vi "Resource Editor.vi"(7 "Load from Initial Path (F)":bool, 10 "Initial Resources":T1, 11 "Path":path) -> (2 "Final Resources":T1)   [LabVIEW 2023]
doc: "Edits several types of LabVIEW files at a low level, including VI's.\n\nCan also be used as a dialog subVI for editing resource clusters."
uses:
  Resource Manipulation/Resource Array.ctl
  Resource Manipulation/Resource.ctl
  CTLs/Resource Editor Internal Commands Enum.ctl
  Resource Manipulation.lvlib
panel:
  out "Initial Resources 2":T1
  in  "Delete":bool
  in  "Add":bool
  in  "Name":string
  in  "Type":string
  in  "ID":i32
  in  "Export":bool
  in  "Import":bool
  in  "Paste":bool
  in  "Copy":bool
  in  "XML":bool
  in  "Fix MD5":bool
  in  "File type":string
  in  "Data":string
  in  "Hex view":bool
  in  "Save":bool
  in  "Load":bool
  in  "Resources":i32(listbox)=-1
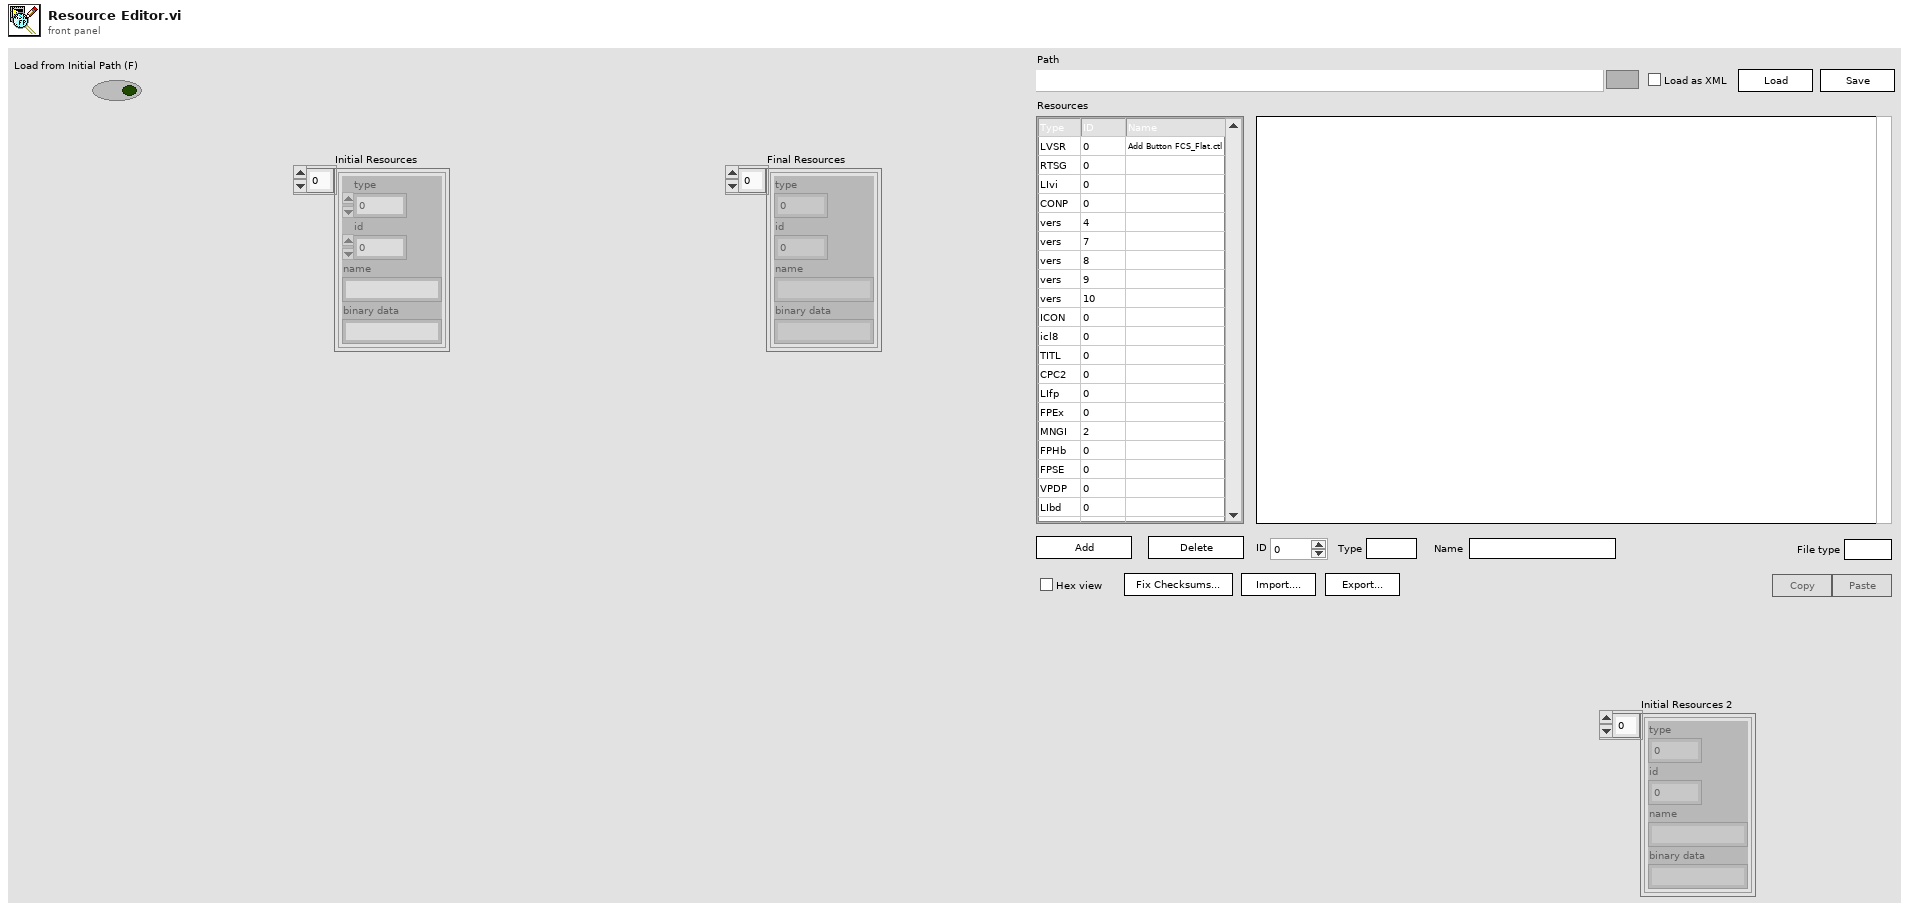
[diagram p1: front panel]
types:
  T1 = typedef "Resource Manipulation.lvlib/Resource Array.ctl" = T2[]
  T2 = typedef "Resource Manipulation.lvlib/Resource.ctl" = cluster{"type":u32, "id":i32, "name":string, "binary data":string}
  T3 = typedef "Resource Editor Internal Commands Enum.ctl" = enum16{"Refresh Resource List", "Load from Path"}
  T4 = enum8{"Enabled", "Disabled", "Disabled and Grayed Out"}
  T5 = enum16{"Left Button", "Center Button", "Right Button", "Window Close"}
  T6 = enum16{"open", "replace", "create", "open or create", "replace or create", "replace or create with confirmation"}
  T7 = typedef "Resource Manipulation.lvlib/Terminal Counts.ctl" = cluster{"Numbers":u32, "Strings":u32, "Paths":u32}
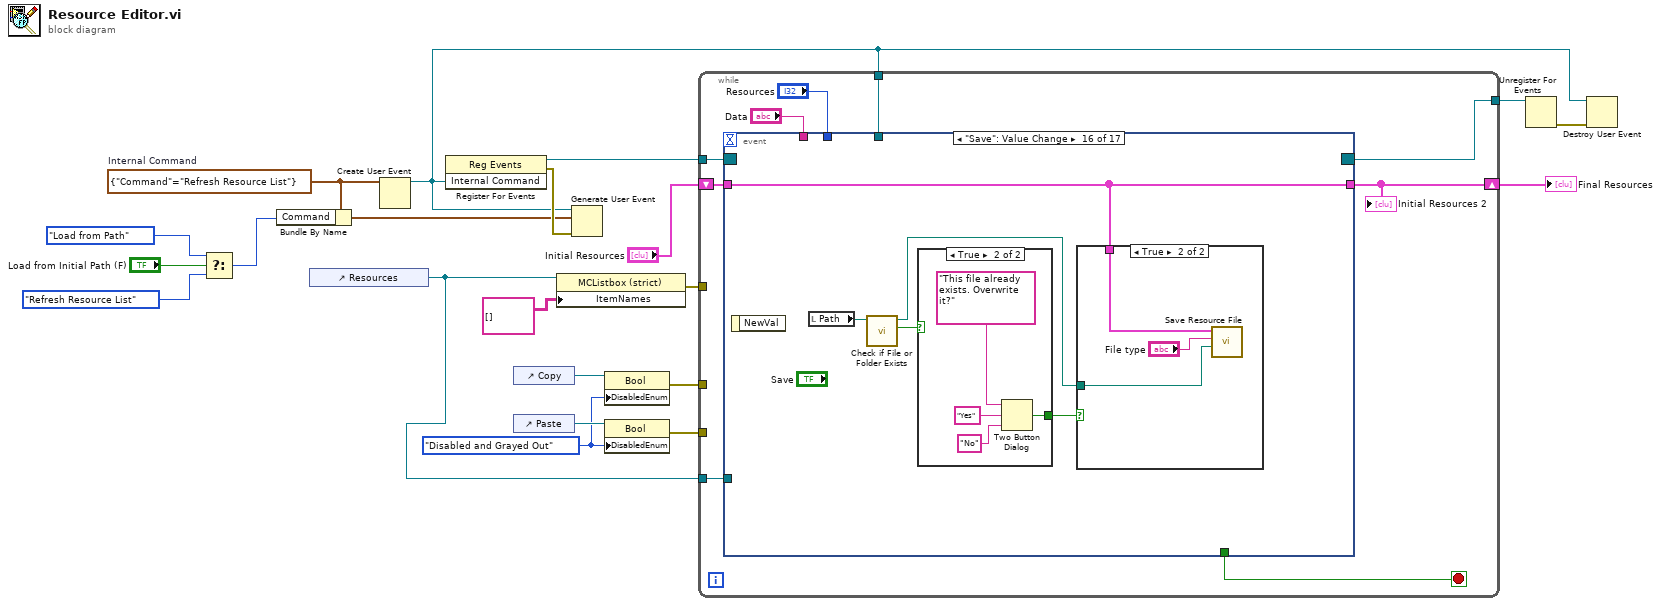
[diagram p0: block diagram]
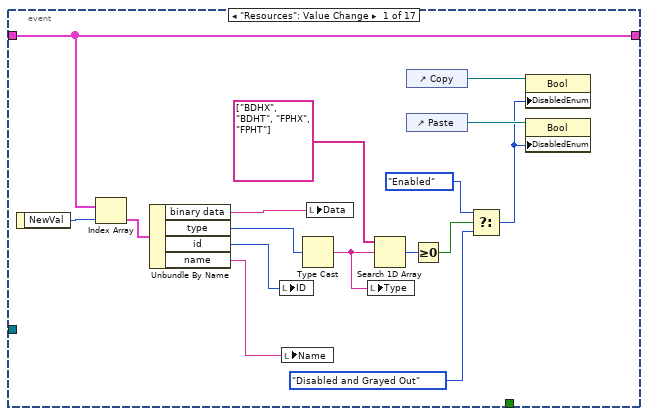
[diagram p2: hidden frame]
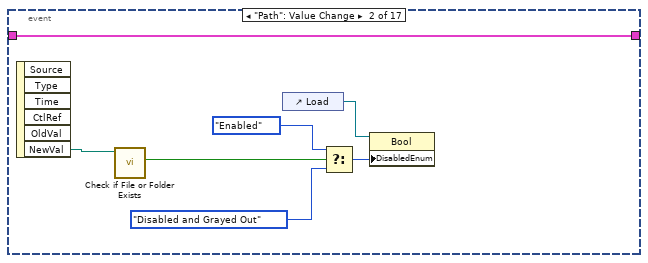
[diagram p3: hidden frame]
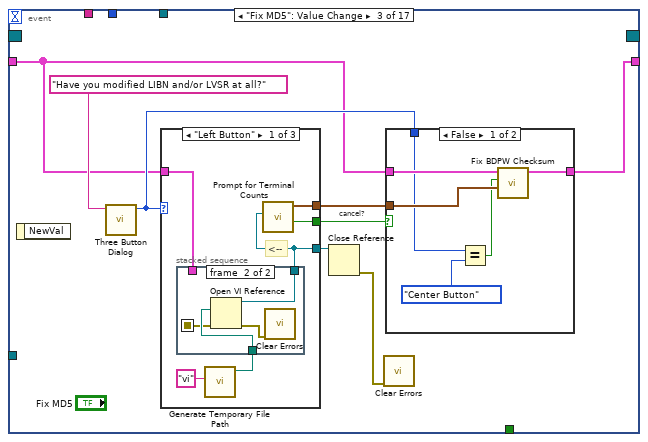
[diagram p4: hidden frame]
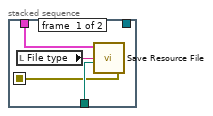
[diagram p5: hidden frame]
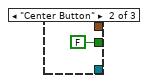
[diagram p6: hidden frame]
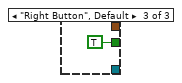
[diagram p7: hidden frame]
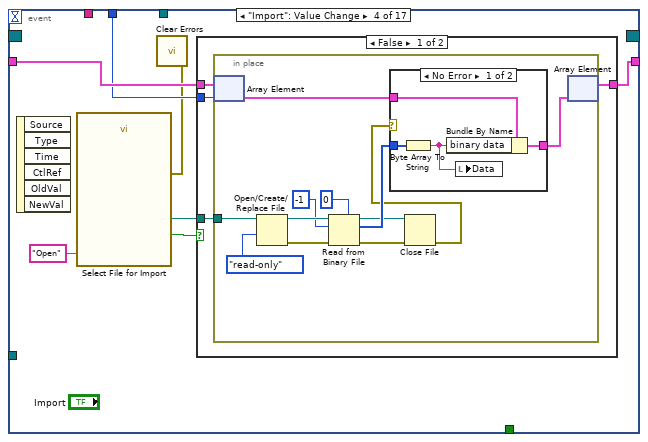
[diagram p9: hidden frame]
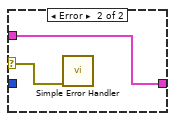
[diagram p10: hidden frame]
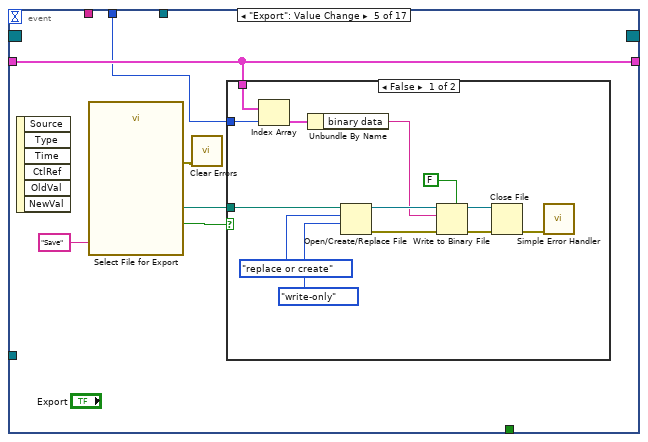
[diagram p12: hidden frame]
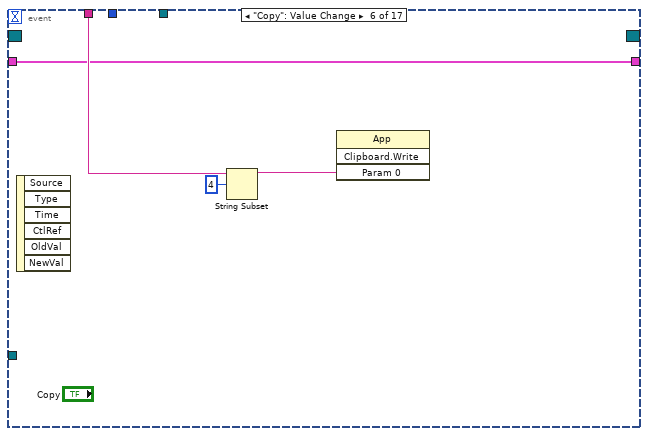
[diagram p14: hidden frame]
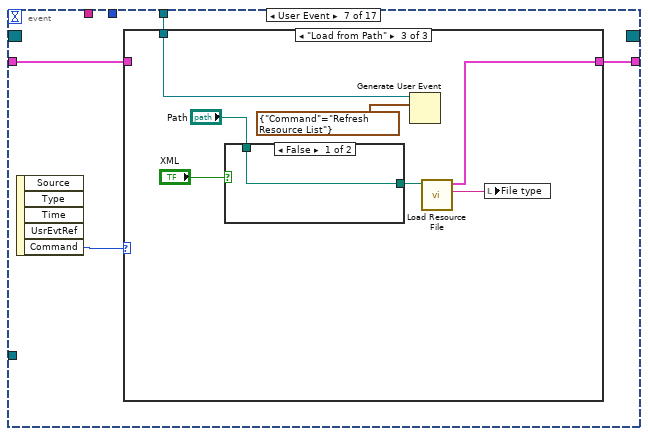
[diagram p15: hidden frame]
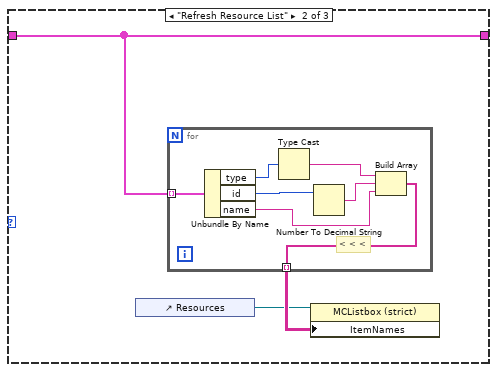
[diagram p17: hidden frame]
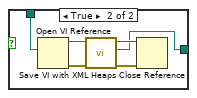
[diagram p18: hidden frame]
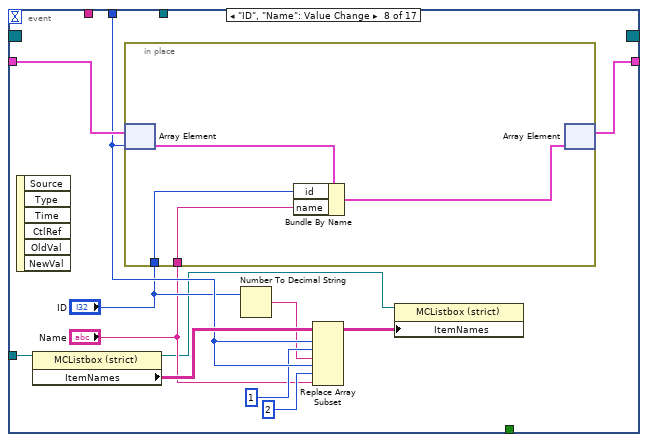
[diagram p19: hidden frame]
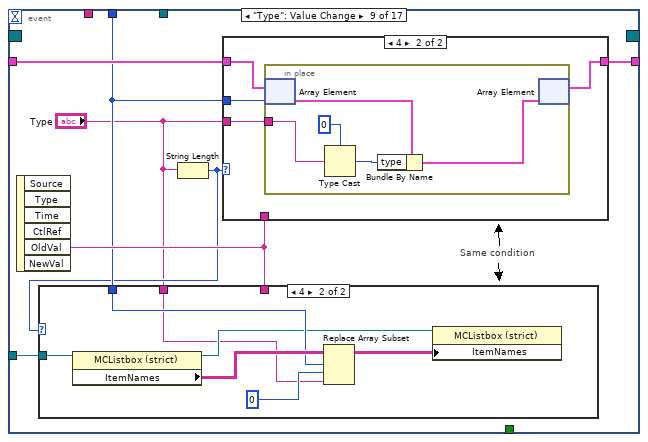
[diagram p20: hidden frame]
diagram:
  w6 = cluster{"Command":T3} {"Command"=enum."Refresh Resource List"}  # Internal Command
  w16 = T4."Disabled and Grayed Out" ("Disabled")
  n1 = Select(t=Resource_Editor_Internal_Commands_Enum."Load from Path" ("Command"), s="Load from Initial Path (F)", f=Resource_Editor_Internal_Commands_Enum."Refresh Resource List" ("Command")) -> (s? t:f=w1:T3)
  n2 = Bundle By Name(cluster=w6, "Command"=w1) -> (w5:cluster{"Command":T3})
  n3 = control-ref of="Resources"() -> (w13:refnum<vi>)
  n4 = Create User Event(user event datatype=w6) -> (user event=w7:refnum<user-event>)  [unwired: 1 in, 1 out]
  n5 = register-events(w7) -> (reference out=w8:refnum<event-registration>, error out=w9:errorcluster)  [unwired: 2 in]
  n6 = control-ref of="Copy"() -> (w18:refnum<vi>)
  n7 = control-ref of="Paste"() -> (w17:refnum<vi>)
  n8 = property class="MCListbox (strict)"(reference=w13, "ItemNames"=string[][] [] ("Item Names")) -> (error out=w20:errorcluster)  [unwired: 1 in, 1 out]
  n9 = Generate User Event(user event=w7, event data cluster=w5, error in=w9) -> ()  [unwired: 1 in, 2 out]
  n10 = property class="Bool"(reference=w18, "DisabledEnum"=w16) -> (error out=w15:errorcluster)  [unwired: 1 in, 1 out]
  n11 = property class="Bool"(reference=w17, "DisabledEnum"=w16) -> (error out=w14:errorcluster)  [unwired: 1 in, 1 out]
  n12 = while {
    shift-right: [w29] -> w12
    shift-left: "Initial Resources" -> [w30]
    tunnel: w20 -> [_]
    tunnel: w15 -> [_]
    tunnel: w14 -> [_]
    tunnel: w13 -> [w25]
    tunnel: w8 -> [w24]
    tunnel: w7 -> [w23]
    tunnel: [w22] -> w11
    stop <- w28 stop-if-true
    n13 = event shown="[15] \"Save\": Value Change" {
      selector: w24 -> [_ _ _ _ _ _ _ _ _ _ _ _ _ _ _ _ _]
      dyn-events: [_ _ _ _ _ _ _ _ _ _ _ _ _ _ _ _ _] -> w22
      timeout: _ -> [_ _ _ _ _ _ _ _ _ _ _ _ _ _ _ _ _]
      tunnel: w30 -> [w44 w47 w57 w91 w120 w136 w139 w178 w189 w216 w232 w241 w246 w253 w260 w265 w274]
      tunnel: [w44 w47 w61 w89 w120 w136 w140 w177 w188 w214 w230 w241 w246 w251 w258 w265 w274] -> w29
      tunnel: [_ _ _ _ _ _ _ _ _ _ _ _ _ _ _ _ w275] -> w28
      tunnel: "Data" -> [_ _ _ _ _ w137 _ _ _ _ _ _ _ _ _ _ _]
      tunnel: "Resources" -> [_ _ _ w90 w117 _ _ w175 w185 w215 w229 _ _ w247 w259 _ _]
      tunnel: w25 -> [_ _ _ _ _ _ _ w168 w187 _ _ _ _ _ _ _ _]
      tunnel: w23 -> [_ _ _ _ _ _ w138 _ _ _ _ _ w244 _ w257 _ _]
      event "Resources": Value Change {
        n14 = event-data() -> ("NewVal"=w46:i32)  [unwired: 1 in]
        n15 = Index Array(array=w44, index=w46) -> (element=w45:T2)
        n16 = Unbundle By Name(w45) -> ("binary data"=w43:string, "type"=w42:u32, "id"=w33:i32, "name"=w32:string)
        n17 = local write "ID"(w33) -> ()
        n18 = local write "Name"(w32) -> ()
        n19 = Type Cast(x=w42) -> (*(type *) &x=w31:string)  [unwired: 1 in]
        n20 = local write "Data"(w43) -> ()
        n21 = local write "Type"(w31) -> ()
        n22 = Search 1D Array(1D array=string[] ["BDHX", "BDHT", "FPHX", "FPHT"], element=w31) -> (index of element=w38:i32)  [unwired: 1 in]
        n23 = control-ref of="Copy"() -> (w40:refnum<vi>)
        n24 = control-ref of="Paste"() -> (w39:refnum<vi>)
        n25 = Greater Or Equal To 0?(x=w38) -> (x >= 0?=w37:bool)
        n26 = Select(t=T4."Enabled" ("Disabled"), s=w37, f=T4."Disabled and Grayed Out" ("Disabled")) -> (s? t:f=w34:T4)
        n27 = property class="Bool"(reference=w40, "DisabledEnum"=w34) -> ()  [unwired: 1 in, 2 out]
        n28 = property class="Bool"(reference=w39, "DisabledEnum"=w34) -> ()  [unwired: 1 in, 2 out]
      }
      event "Path": Value Change {
        n29 = event-data() -> ("NewVal"=w53:path)  [unwired: 1 in, 5 out]
        n30 = call <vilib>:"Check if File or Folder Exists.vi"("path"=w53) -> ("file or folder exists?"=w48:bool)  [unwired: 8 in, 2 out]
        n31 = control-ref of="Load"() -> (w52:refnum<vi>)
        n32 = Select(t=T4."Enabled" ("Disabled"), s=w48, f=T4."Disabled and Grayed Out" ("Disabled")) -> (s? t:f=w49:T4)
        n33 = property class="Bool"(reference=w52, "DisabledEnum"=w49) -> ()  [unwired: 1 in, 2 out]
      }
      event "Fix MD5": Value Change {
        # "cancel?"
        n34 = event-data() -> ()  [unwired: 1 in, 1 out]
        n35 = call <vilib>:"Three Button Dialog.vi"("message"="Have you modified LIBN and/or LVSR at all?") -> ("Which Button?"=w58:T5)  [unwired: 10 in]
        n36 = case shown="\"Left Button\"" w58 {
          tunnel: [w67 FALSE ("Canceled?") TRUE ("Canceled?")] -> w56
          tunnel: [w66 _ _] -> w60
          tunnel: w57 -> [w63 _ _]
          tunnel: [w62 _ _] -> w55
          frame "Left Button" {
            # "<--"
            n37 = call <vilib>:"Generate Temporary File Path.vi"("Temporary File Extension (tmp)"="vi") -> ("Unique Temporary File Path"=w65:path)  [unwired: 9 in, 1 out]
            n38 = stacked-sequence {
              seq-local: [w68 _] -> [_ w72]
              tunnel: w65 -> [w71 w74]
              tunnel: w63 -> [w70 _]
              tunnel: [_ w75] -> w62
              frame #0 {
                n39 = local read "File type"() -> (w69:string)
                n40 = call "Save Resource File.vi"("Path"=w71, "File type"=w69, "Resources"=w70) -> ("error out"=w68:errorcluster)  [unwired: 8 in]
              }
              frame #1 {
                n41 = Open VI Reference(vi path=w74, error in (no error)=w72) -> (vi reference=w75:refnum<vi>, error out=w73:errorcluster)  [unwired: 4 in]
                n42 = call <vilib>:"Clear Errors.vi"("error in (no error)"=w73) -> ()  [unwired: 5 in, 2 out]
              }
            }
            n43 = call "Prompt for Terminal Counts.vi"("Reference VI"=w62) -> ("Canceled?"=w67:bool, "Terminal Counts"=w66:T7)  [unwired: 9 in]
          }
          frame "Center Button" {
          }
          frame "Right Button", Default {
          }
        }
        n44 = Close Reference(reference=w55) -> (error out=w54:errorcluster)  [unwired: 1 in]
        n45 = call <vilib>:"Clear Errors.vi"("error in (no error)"=w54) -> ()  [unwired: 5 in, 2 out]
        n46 = case shown="False" w56 {
          tunnel: w57 -> [w83 w84]
          tunnel: [w82 w84] -> w61
          tunnel: w60 -> [w81 _]
          tunnel: w58 -> [w79 _]
          frame False {
            n47 = Equal?(x=w79, y=T5."Center Button" ("Which Button?")) -> (x = y?=w78:bool)
            n48 = call "Fix BDPW Checksum.vi"("Terminal Counts"=w81, "Only fix 3rd hash (F)"=w78, "Resources in"=w83) -> ("Resources out"=w82:T1)  [unwired: 8 in]
          }
          frame True {
          }
        }
      }
      event "Import": Value Change {
        n49 = event-data() -> ()  [unwired: 1 in, 6 out]
        n50 = call "Select File for Import"("button label"="Open") -> ("selected path"=w87:path, "cancelled"=w88:bool, "error out"=w85:errorcluster)  [unwired: 11 in, 1 out]
        n51 = call <vilib>:"Clear Errors.vi"("error in (no error)"=w85) -> ()  [unwired: 5 in, 2 out]
        n52 = case shown="False" w88 {
          tunnel: w91 -> [w95 w114]
          tunnel: w90 -> [w94 _]
          tunnel: [w93 w114] -> w89
          tunnel: w87 -> [w92 _]
          frame False {
            n53 = in-place {
              in-place-border: w92 -> [w107]
              n54 = in-place-array #1(w95, w94) -> (w101:T2)
              n55 = Open/Create/Replace File(file path (use dialog)=w107, access (0:read/write)=enum16{"read/write", "read-only", "write-only"}."read-only") -> (refnum out=w105:refnum<file>, error out=w102:errorcluster)  [unwired: 4 in, 1 out]
              n56 = Read from Binary File(5:u8 0, 8:w102, 10:-1 ("count (1)"), 11:w105) -> (0:w97:errorcluster, 2:w100:u8[], 3:w98:refnum<file>)  [unwired: 2 in, 1 out]
              n57 = Close File(refnum=w98, error in=w97) -> (error out=w96:errorcluster)  [unwired: 1 out]
              n58 = case shown="No Error" w96 {
                selector: w96 -> [_ w112]
                tunnel: w101 -> [w111 w113]
                tunnel: w100 -> [w110 _]
                tunnel: [w109 w113] -> w99
                frame No Error {
                  n59 = Byte Array To String(unsigned byte array=w110) -> (string=w108:string)
                  n60 = Bundle By Name(cluster=w111, "binary data"=w108) -> (w109:T2)
                  n61 = local write "Data"(w108) -> ()
                }
                frame Error {
                  n62 = call <vilib>:"Simple Error Handler.vi"("error in (no error)"=w112) -> ()  [unwired: 4 in, 5 out]
                }
              }
              n63 = in-place-array #1(w99) -> (w93:T1)  [unwired: 1 out]
            }
          }
          frame True {
          }
        }
      }
      event "Export": Value Change {
        n64 = event-data() -> ()  [unwired: 1 in, 6 out]
        n65 = call "Select File for Export"("button label"="Save") -> ("selected path"=w118:path, "cancelled"=w119:bool, "error out"=w115:errorcluster)  [unwired: 11 in, 1 out]
        n66 = call <vilib>:"Clear Errors.vi"("error in (no error)"=w115) -> ()  [unwired: 5 in, 2 out]
        n67 = case shown="False" w119 {
          tunnel: w120 -> [w128 _]
          tunnel: w118 -> [w133 _]
          tunnel: w117 -> [w127 _]
          frame False {
            n68 = Index Array(array=w128, index=w127) -> (element=w126:T2)
            n69 = Unbundle By Name(w126) -> ("binary data"=w125:string)
            n70 = Open/Create/Replace File(file path (use dialog)=w133, operation (0:open)=T6."replace or create", access (0:read/write)=enum16{"read/write", "read-only", "write-only"}."write-only") -> (refnum out=w129:refnum<file>, error out=w122:errorcluster)  [unwired: 3 in, 1 out]
            n71 = Write to Binary File(file (use dialog)=w129, data=w125, error in=w122, 5:FALSE ("prepend array or string size? (T)")) -> (refnum out=w123:refnum<file>, error out=w124:errorcluster)  [unwired: 2 in, 1 out]
            n72 = Close File(refnum=w123, error in=w124) -> (error out=w121:errorcluster)  [unwired: 1 out]
            n73 = call <vilib>:"Simple Error Handler.vi"("error in (no error)"=w121) -> ()  [unwired: 4 in, 5 out]
          }
          frame True {
          }
        }
      }
      event "Copy": Value Change {
        n74 = event-data() -> ()  [unwired: 1 in, 6 out]
        n75 = String Subset(string=w137, offset (0)=4) -> (substring=w135:string)  [unwired: 1 in]
        n76 = invoke class="App" method="Clipboard.Write"("Param 0"=w135) -> ()  [unwired: 3 in, 4 out]
      }
      event User Event {
        n77 = event-data() -> ("Command"=w141:T3)  [unwired: 1 in, 4 out]
        n78 = case shown="\"Load from Path\"" w141 {
          tunnel: [w142 w144 w155] -> w140
          tunnel: w139 -> [w142 w144 _]
          tunnel: w138 -> [_ _ w153]
          frame Default {
          }
          frame "Refresh Resource List" {
            n79 = control-ref of="Resources"() -> (w143:refnum<vi>)
            n80 = for {
              tunnel: [w152] -> w145 mode=indexing
              tunnel: w144 -> [w148] mode=indexing
              # "< < <"
              n81 = Unbundle By Name(w148) -> ("type"=w151:u32, "id"=w147:i32, "name"=w146:string)
              n82 = Type Cast(x=w151) -> (*(type *) &x=w149:string)  [unwired: 1 in]
              n83 = Number To Decimal String(number=w147) -> (decimal integer string=w150:string)  [unwired: 1 in]
              n84 = Build Array(w149, w150, w146) -> (w152:string[])
            }
            n85 = property class="MCListbox (strict)"(reference=w143, "ItemNames"=w145) -> ()  [unwired: 1 in, 2 out]
          }
          frame "Load from Path" {
            n86 = case shown="False" "XML" {
              tunnel: "Path" -> [w160 w166]
              tunnel: [w160 w161] -> w158
              frame False {
              }
              frame True {
                n87 = Open VI Reference(vi path=w166) -> (vi reference=w165:refnum<vi>, error out=w164:errorcluster)  [unwired: 5 in]
                n88 = call "Save VI with XML Heaps.vi"("error in (no error)"=w164, "VI Refnum In"=w165) -> ("error out"=w163:errorcluster, "VI Path out"=w161:path, "VI Refnum Out"=w162:refnum<vi>)  [unwired: 7 in]
                n89 = Close Reference(reference=w162, error in (no error)=w163) -> ()  [unwired: 1 out]
              }
            }
            n90 = Generate User Event(user event=w153, event data cluster=cluster{"Command":T3} {"Command"=enum."Refresh Resource List"} ("event data")) -> ()  [unwired: 2 in, 2 out]
            n91 = call "Load Resource File.vi"("Resource File"=w158) -> ("File Type"=w154:string, "Resources"=w155:T1)  [unwired: 8 in, 1 out]
            n92 = local write "File type"(w154) -> ()
          }
        }
      }
      event "ID", "Name": Value Change {
        n93 = event-data() -> ()  [unwired: 1 in, 6 out]
        n94 = property class="MCListbox (strict)"(reference=w168) -> (reference out=w167:refnum<vi>, "ItemNames"=w176:string[][])  [unwired: 1 in, 1 out]
        n95 = in-place {
          in-place-border: "ID" -> [w180]
          in-place-border: "Name" -> [w179]
          n96 = in-place-array #2(w178, w175) -> (w182:T2)
          n97 = Bundle By Name(cluster=w182, "id"=w180, "name"=w179) -> (w181:T2)
          n98 = in-place-array #2(w181) -> (w177:T1)  [unwired: 1 out]
        }
        n99 = Number To Decimal String(number="ID") -> (decimal integer string=w171:string)  [unwired: 1 in]
        n100 = Replace Array Subset(array=w176, new element #1=w171, index (row) #1=w175, index (col) #1=1, new element #2="Name", index (row) #2=w175, index (col) #2=2) -> (w169:string[][])
        n101 = property class="MCListbox (strict)"(reference=w167, "ItemNames"=w169) -> ()  [unwired: 1 in, 2 out]
      }
      event "Type": Value Change {
        # "Same condition"
        n102 = event-data() -> ("OldVal"=w186:string)  [unwired: 1 in, 5 out]
        n103 = String Length(string="Type") -> (length=w184:i32)
        n104 = case shown="4" w184 {
          tunnel: w187 -> [_ w196]
          tunnel: w186 -> [_ _]
          tunnel: w185 -> [_ w194]
          tunnel: "Type" -> [_ w190]
          frame Default {
          }
          frame 4 {
            n105 = property class="MCListbox (strict)"(reference=w196) -> (reference out=w191:refnum<vi>, "ItemNames"=w195:string[][])  [unwired: 1 in, 1 out]
            n106 = Replace Array Subset(array=w195, new element=w190, index (row)=w194, index (col)=0) -> (w192:string[][])
            n107 = property class="MCListbox (strict)"(reference=w191, "ItemNames"=w192) -> ()  [unwired: 1 in, 2 out]
          }
        }
        n108 = case shown="4" w184 {
          tunnel: "Type" -> [_ w200]
          tunnel: w189 -> [w198 w202]
          tunnel: w185 -> [_ w201]
          tunnel: [w198 w199] -> w188
          tunnel: w186 -> [w197 _]
          frame Default {
            n109 = local write "Type"(w197) -> ()
            n110 = call <vilib>:"Beep.vi"() -> ()  [unwired: 12 in]
          }
          frame 4 {
            n111 = in-place {
              in-place-border: w200 -> [w206]
              n112 = in-place-array #3(w202, w201) -> (w207:T2)
              n113 = Type Cast(type=u32 0, x=w206) -> (*(type *) &x=w204:u32)
              n114 = Bundle By Name(cluster=w207, "type"=w204) -> (w203:T2)
              n115 = in-place-array #3(w203) -> (w199:T1)  [unwired: 1 out]
            }
          }
        }
      }
      event "Paste": Value Change {
        # "< < <"
        n116 = event-data() -> ()  [unwired: 1 in, 6 out]
        n117 = invoke class="App" method="Clipboard.Read"() -> (error out=w217:errorcluster, "Read Clipbrd"=w209:string)  [unwired: 3 in, 1 out]
        n118 = call "Is Big Endian.vi"() -> ("big endian"=w213:bool)
        n119 = String Length(string=w209) -> (length=w211:i32)
        n120 = Type Cast(x=w211) -> (*(type *) &x=w212:string)  [unwired: 1 in]
        n121 = case shown="True" w213 {
          tunnel: w212 -> [w218 w220]
          tunnel: [w218 w219] -> w208
          frame False {
          }
          frame True {
            n122 = Reverse String(1:w220) -> (0:w219:string)
          }
        }
        n123 = Concatenate Strings(w208, w209) -> (w210:string)
        n124 = case shown="Error" w217 {
          tunnel: w210 -> [w222 _]
          tunnel: w216 -> [w223 w228]
          tunnel: w215 -> [w224 _]
          tunnel: [w221 w228] -> w214
          frame No Error {
            n125 = in-place {
              in-place-border: w222 -> [w225]
              n126 = in-place-array #4(w223, w224) -> (w226:T2)
              n127 = local write "Data"(w225) -> ()
              n128 = Bundle By Name(cluster=w226, "binary data"=w225) -> (w227:T2)
              n129 = in-place-array #4(w227) -> (w221:T1)  [unwired: 1 out]
            }
          }
          frame Error {
          }
        }
      }
      event "Data": Value Change {
        n130 = event-data() -> ("NewVal"=w231:string)  [unwired: 1 in]
        n131 = in-place {
          in-place-border: w231 -> [w234]
          n132 = in-place-array #5(w232, w229) -> (w235:T2)
          n133 = Bundle By Name(cluster=w235, "binary data"=w234) -> (w233:T2)
          n134 = in-place-array #5(w233) -> (w230:T1)  [unwired: 1 out]
        }
      }
      event "Hex view": Value Change {
        n135 = event-data() -> ()  [unwired: 1 in, 1 out]
        n136 = Select(t=u32 3 ("Display Style"), s="Hex view", f=u32 0 ("Display Style")) -> (s? t:f=w237:u32)
        n137 = control-ref of="Data"() -> (w240:refnum<vi>)
        n138 = property class="Str"(reference=w240, "Display Style"=w237) -> ()  [unwired: 1 in, 2 out]
      }
      event "Load": Value Change {
        n139 = event-data() -> ()  [unwired: 1 in, 1 out]
        n140 = control-ref of="Resources"() -> (w243:refnum<vi>)
        n141 = Generate User Event(user event=w244, event data cluster=cluster{"Command":T3} {"Command"=enum."Load from Path"}) -> ()  [unwired: 2 in, 2 out]
        n142 = property class="MCListbox (strict)"(reference=w243, "Val(Sgnl)"=0 ("Value (Signaling)")) -> ()  [unwired: 1 in, 2 out]
      }
      event "Add": Value Change {
        n143 = event-data() -> ()  [unwired: 1 in, 6 out]
        n144 = control-ref of="Resources"() -> (w255:refnum<vi>)
        n145 = Insert Into Array(array=w253, index=w247, new element=T2 {"type"=1315272530, "id"=0, "name"="", "binary data"=""} ("element")) -> (w251:T1)
        n146 = property class="MCListbox (strict)"(reference=w255) -> (reference out=w254:refnum<vi>, "ItemNames"=w250:string[][])  [unwired: 1 in, 1 out]
        n147 = Insert Into Array(array=w250, index (row)=w247, new element=string[] ["NewR", "0", ""]) -> (w249:string[][])  [unwired: 1 in]
        n148 = property class="MCListbox (strict)"(reference=w254, "ItemNames"=w249, "Val(Sgnl)"=w247) -> ()  [unwired: 1 in, 2 out]
      }
      event "Delete": Value Change {
        n149 = event-data() -> ()  [unwired: 1 in, 6 out]
        n150 = Delete From Array(array=w260, index=w259) -> (array with subset deleted=w258:T1)  [unwired: 1 in, 1 out]
        n151 = Generate User Event(user event=w257, event data cluster=cluster{"Command":T3} {"Command"=enum."Refresh Resource List"} ("event data")) -> ()  [unwired: 2 in, 2 out]
      }
      event "Save": Value Change {
        n152 = event-data() -> ()  [unwired: 1 in, 1 out]
        n153 = local read "Path"() -> (w261:path)
        n154 = call <vilib>:"Check if File or Folder Exists.vi"("path"=w261) -> ("file or folder exists?"=w264:bool, "dup path"=w262:path)  [unwired: 8 in, 1 out]
        n155 = case shown="True" w264 {
          tunnel: [TRUE ("T button?") w271] -> w263
          frame False {
          }
          frame True {
            n156 = Two Button Dialog(message="This file already exists. Overwrite it?", 1:"No", 2:"Yes" ("T button name (\"OK\")")) -> (T button?=w271:bool)
          }
        }
        n157 = case shown="True" w263 {
          tunnel: w265 -> [_ w268]
          tunnel: w262 -> [_ w266]
          frame False {
          }
          frame True {
            n158 = call "Save Resource File.vi"("Path"=w266, "File type"="File type", "Resources"=w268) -> ()  [unwired: 8 in, 1 out]
          }
        }
      }
      event Panel Close? {
        w275 = TRUE ("Discard?")
        n159 = event-data() -> ()  [unwired: 1 in, 1 out]
        n160 = event-data("Discard?"=w275) -> ()  [unwired: 1 in, 1 out]
      }
    }
    "Initial Resources 2" <- w29
  }
  "Final Resources" <- w12
  n161 = Unregister For Events(event registration refnum=w11) -> (error out=w10:errorcluster)  [unwired: 1 in]
  n162 = Destroy User Event(user event=w7, error in=w10) -> ()  [unwired: 1 out]
